vi "get_targets.vi"(2 "error in (no error)":errorcluster, 3 "Listen Port":u16=5311, 4 "Remote Server Port":u16=5310, 5 "Remote Server Address":string="us-aus-rtweb1") -> (0 "error out":errorcluster, 1 "Target Array":T1[](array[typedef]))   [LabVIEW 2011]
uses:
  TCPdata.ctl
  TargetData.ctl
  CommonTargetData.ctl
panel:
  in  "Target Array Type":T3(array[cluster])
  in  "Cluster":T4
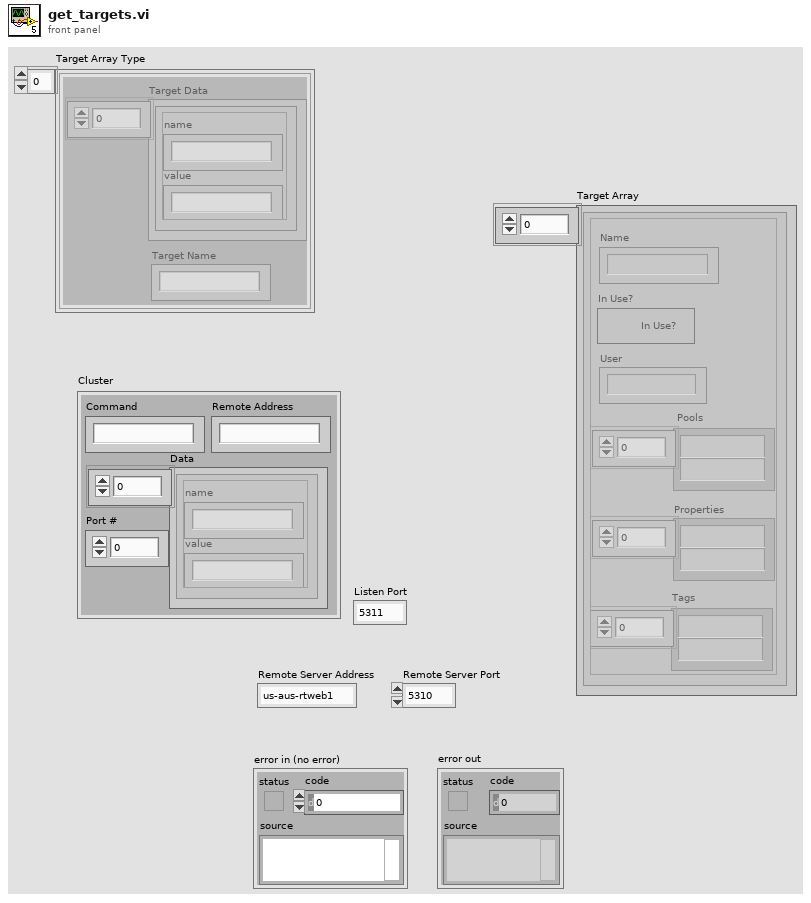
[diagram p1: front panel]
types:
  T1 = typedef "CommonTargetData.ctl" = cluster{"Name":string, "In Use?":bool, "User":string, " Pools":string[], "Tags":string[], "Properties":string[]}
  T2 = typedef "TargetData.ctl" = cluster{"name":string, "value":string}[]
  T3 = cluster{"Target Data":T2, "Target Name":string}[]
  T4 = typedef "TCPdata.ctl" = cluster{"Data":T2, "Command":string, "Remote Address":string, "Port #":u16}
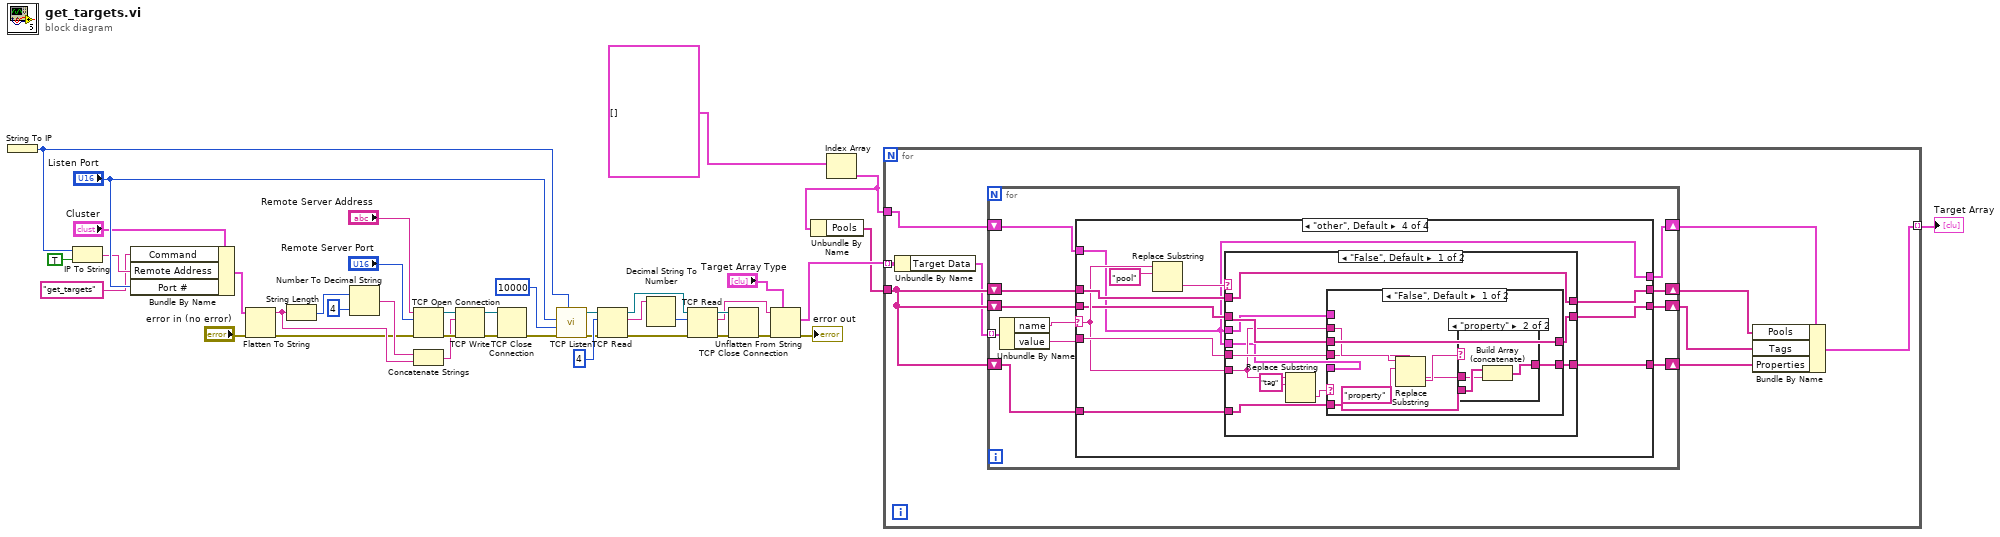
[diagram p0: block diagram]
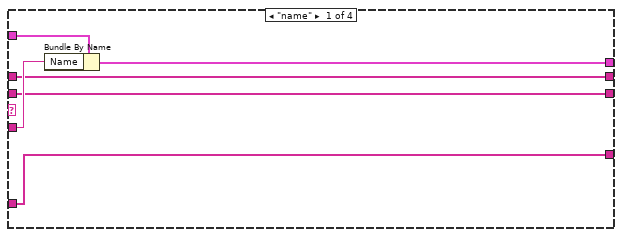
[diagram p2: hidden frame]
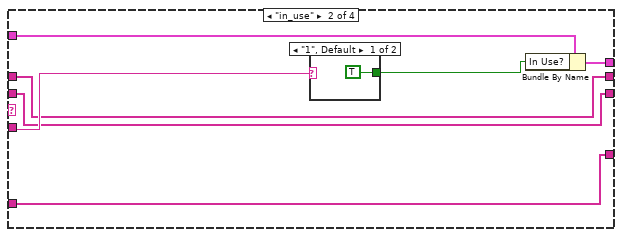
[diagram p3: hidden frame]
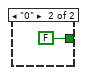
[diagram p4: hidden frame]
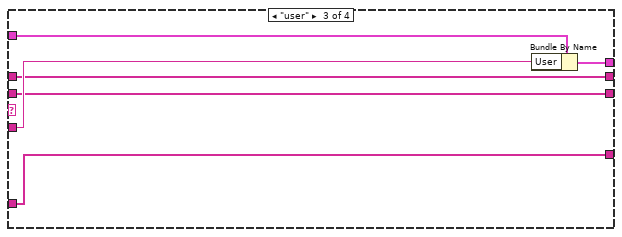
[diagram p5: hidden frame]
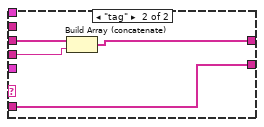
[diagram p7: hidden frame]
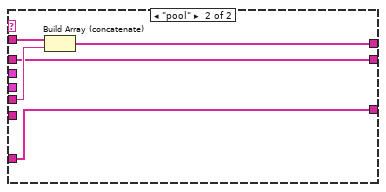
[diagram p8: hidden frame]
diagram:
  n1 = String To IP() -> (0:w26:u32)  [unwired: 1 in]
  n2 = IP To String(1:TRUE ("dot notation? (F)"), 2:w26) -> (0:w28:string)
  n3 = Bundle By Name(cluster="Cluster", "Command"="get_targets", "Remote Address"=w28, "Port #"="Listen Port") -> (w8:T4)
  n4 = Flatten To String(anything=w8, error in (no error)="error in (no error)") -> (data string=w21:string, error out=w19:errorcluster)  [unwired: 2 in, 1 out]
  n5 = String Length(string=w21) -> (length=w24:i32)
  n6 = Number To Decimal String(number=w24, width (-)=i16 4) -> (decimal integer string=w23:string)
  n7 = TCP Open Connection(address="Remote Server Address", remote port or service name="Remote Server Port", error in (no error)=w19) -> (connection ID=w40:refnum<k5>, error out=w39:errorcluster)  [unwired: 2 out]
  n8 = Concatenate Strings(w23, w21) -> (w25:string)
  n9 = TCP Write(connection ID=w40, data in=w25, error in (no error)=w39) -> (connection ID out=w37:refnum<k5>, error out=w38:errorcluster)  [unwired: 2 out]
  n10 = TCP Close Connection(connection ID=w37, error in (no error)=w38) -> (error out=w31:errorcluster)  [unwired: 2 out]
  n11 = call <vilib>:"TCP Listen.vi"("net address"=w26, "error in (no error)"=w31, "timeout ms (wait forever: -1)"=10000, "port"="Listen Port") -> ("error out"=w16:errorcluster, "connection ID"=w14:refnum<k5>)  [unwired: 3 in, 3 out]
  n12 = TCP Read(connection ID=w14, bytes to read=4, error in (no error)=w16) -> (connection ID out=w13:refnum<k5>, data out=w17:string, error out=w15:errorcluster)  [unwired: 1 in, 1 out]
  n13 = Decimal String To Number(string=w17) -> (number=w12:i32)  [unwired: 2 in, 1 out]
  n14 = TCP Read(connection ID=w13, bytes to read=w12, error in (no error)=w15) -> (connection ID out=w34:refnum<k5>, data out=w10:string, error out=w32:errorcluster)  [unwired: 1 in, 1 out]
  n15 = TCP Close Connection(connection ID=w34, error in (no error)=w32) -> (error out=w11:errorcluster)  [unwired: 2 out]
  n16 = Unflatten From String(type="Target Array Type", binary string=w10, error in (no error)=w11) -> (value=w5:T3, error out=→"error out":errorcluster)  [unwired: 2 in, 1 out]
  n17 = Index Array(array=T1[] [] ("Target Array")) -> (element=w3:T1)  [unwired: 1 in]
  n18 = Unbundle By Name(w3) -> ("Pools"=w2:string[])
  n19 = for {
    tunnel: w5 -> [w42] mode=indexing
    tunnel: w3 -> [w49]
    tunnel: [w43] -> w4 mode=indexing
    tunnel: w2 -> [w48]
    n20 = Unbundle By Name(w42) -> ("Target Data"=w41:T2)
    n21 = for {
      shift-right: [w59] -> w47
      shift-left: w49 -> [w60]
      shift-right: [w55] -> w45
      shift-left: w48 -> [w57]
      shift-right: [w56] -> w46
      shift-left: w48 -> [w58]
      shift-right: [w53] -> w44
      shift-left: w48 -> [w54]
      tunnel: w41 -> [w52] mode=indexing
      n22 = Unbundle By Name(w52) -> ("name"=w51:string, "value"=w50:string)
      n23 = case shown="\"other\", Default" w51 {
        selector: w51 -> [_ _ _ w88]
        tunnel: w50 -> [w64 w71 w79 w90]
        tunnel: w60 -> [w66 w73 w81 w84]
        tunnel: [w65 w72 w80 w84] -> w59
        tunnel: w58 -> [w63 w68 w77 w92]
        tunnel: w57 -> [w62 w69 w78 w86]
        tunnel: [w63 w68 w77 w91] -> w56
        tunnel: [w62 w69 w78 w85] -> w55
        tunnel: w54 -> [w61 w67 w76 w83]
        tunnel: [w61 w67 w76 w82] -> w53
        frame "name" {
          n24 = Bundle By Name(cluster=w66, "Name"=w64) -> (w65:T1)
        }
        frame "in_use" {
          n25 = case shown="\"1\", Default" w71 {
            tunnel: [TRUE ("In Use?") FALSE ("In Use?")] -> w70
            frame "1", Default {
            }
            frame "0" {
            }
          }
          n26 = Bundle By Name(cluster=w73, "In Use?"=w70) -> (w72:T1)
        }
        frame "user" {
          n27 = Bundle By Name(cluster=w81, "User"=w79) -> (w80:T1)
        }
        frame "other", Default {
          n28 = Replace Substring(4:"pool" ("substring (\"\")"), 5:w88) -> (0:w87:string)  [unwired: 2 in, 1 out]
          n29 = case shown="\"False\", Default" w87 {
            tunnel: w92 -> [w103 w123]
            tunnel: [w103 w122] -> w91
            tunnel: w90 -> [w100 w121]
            tunnel: w88 -> [w96 _]
            tunnel: w86 -> [w99 w120]
            tunnel: [w98 w120] -> w85
            tunnel: w84 -> [w97 _]
            tunnel: w84 -> [w95 _]
            tunnel: w83 -> [w94 w119]
            tunnel: [w93 w119] -> w82
            frame "False", Default {
              n30 = Replace Substring(4:"tag" ("substring (\"\")"), 5:w96) -> (0:w101:string)  [unwired: 2 in, 1 out]
              n31 = case shown="\"False\", Default" w101 {
                tunnel: w100 -> [w105 w117]
                tunnel: w99 -> [w110 w118]
                tunnel: [w110 w116] -> w98
                tunnel: w97 -> [_ _]
                tunnel: w96 -> [w106 _]
                tunnel: w95 -> [_ _]
                tunnel: w94 -> [w107 w115]
                tunnel: [w104 w115] -> w93
                frame "False", Default {
                  n32 = Replace Substring(4:"property" ("substring (\"\")"), 5:w106) -> (0:w108:string)  [unwired: 2 in, 1 out]
                  n33 = case shown="\"property\"" w108 {
                    tunnel: w107 -> [w111 w114]
                    tunnel: w105 -> [_ w113]
                    tunnel: [w111 w112] -> w104
                    frame "False", Default {
                    }
                    frame "property" {
                      n34 = Build Array (concatenate)(w114, w113) -> (w112:string[])
                    }
                  }
                }
                frame "tag" {
                  n35 = Build Array (concatenate)(w118, w117) -> (w116:string[])
                }
              }
            }
            frame "pool" {
              n36 = Build Array (concatenate)(w123, w121) -> (w122:string[])
            }
          }
        }
      }
    }
    n37 = Bundle By Name(cluster=w47, "Pools"=w46, "Tags"=w45, "Properties"=w44) -> (w43:T1)
  }
  "Target Array" <- w4
